vi "MakeMatlabExperiment.vi"(8 "error in":errorcluster, 11 "experimentFilepath":path) -> (0 "error out":errorcluster, 1 "erros?":bool, 2 "errors":string, 3 "ExpID":string)   [LabVIEW 2017]
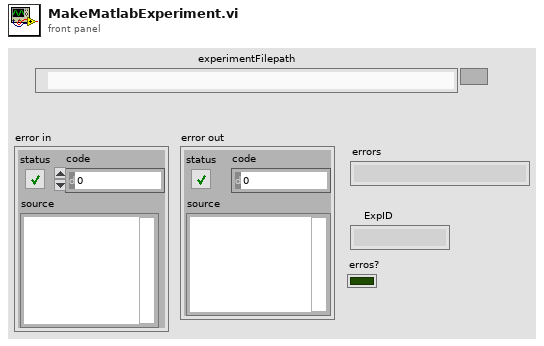
[diagram p1: front panel]
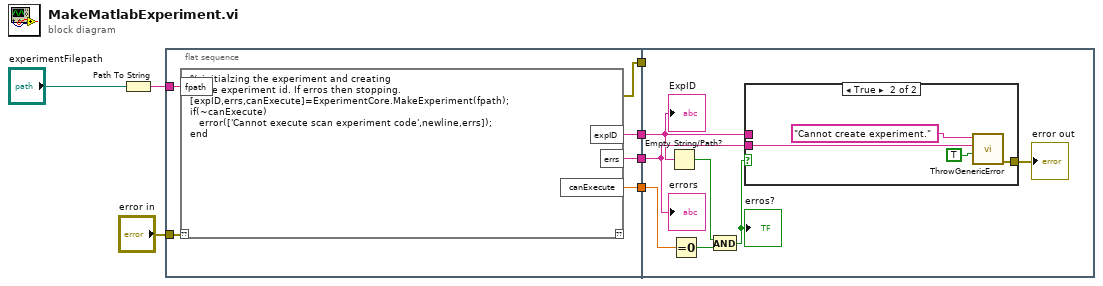
[diagram p0: block diagram]
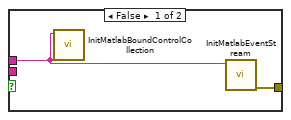
[diagram p2: hidden frame]
diagram:
  n1 = Path To String(path="experimentFilepath") -> (string=w7:string)
  n2 = flat-sequence {
    tunnel: w7 -> [w13]
    tunnel: "error in" -> [w11]
    tunnel: [w12] -> w4
    tunnel: [w10] -> w3
    tunnel: [w9] -> w2
    tunnel: [w8] -> w1
    tunnel: w4 -> [w16]
    tunnel: w3 -> [w20]
    tunnel: w2 -> [_]
    tunnel: w1 -> [w18]
    frame #0 {
      n3 = script code="% initialzing the experiment and creating\n% the experiment id. If erros then stopping.\n[expID,errs,canExecute]=ExperimentCore.MakeExperiment(fpath);\nif(~canExecute)\n   error(['Cannot execute scan experiment code',newline,errs]);\nend"("??"=w11, "fpath"=w13) -> ("??"=w9:errorcluster, "expID"=w8:string, "errs"=w10:string, "canExecute"=w12:dbl)
    }
    frame #1 {
      n4 = Empty String/Path?(string/path=w18) -> (empty?=w14:bool)
      n5 = Equal To 0?(x=w16) -> (x = 0?=w15:bool)
      n6 = And(x=w14, y=w15) -> (x .and. y?=w17:bool)
      "erros?" <- w17
      n7 = case shown="True" w17 {
        tunnel: w20 -> [_ w25]
        tunnel: w18 -> [w21 _]
        tunnel: [w22 w24] -> w19
        frame False {
          n8 = call "InitMatlabBoundControlCollection.vi"("ExpID"=w21) -> ()  [unwired: 10 in, 1 out]
          n9 = call "InitMatlabEventStream.vi"("ExpID"=w21) -> ("error out"=w22:errorcluster)  [unwired: 10 in]
        }
        frame True {
          n10 = call "ThrowGenericError.vi"("Invoke?"=TRUE, "Error info"=w25, "TheError"="Cannot create experiment.") -> ("error out"=w24:errorcluster)  [unwired: 8 in]
        }
      }
      "error out" <- w19
      "ExpID" <- w18
      "errors" <- w20
    }
  }
